vi "Measurement Logic.vi"() -> ()   [LabVIEW 2021, in "Waveform Mode_Channel Ganging.lvlib"]
uses:
  Waveform Mode_Channel Ganging.lvlib
  <vilib>/Plug-In SDKs/Measurements/Measure Call Context/Measure Call Context.lvclass
  Measurement Results.ctl
  Measurement Configuration.ctl
  shared/Ganging/controls/Power ON-Ganging.ctl
  shared/Single/controls/Power ON-Single.ctl
panel:
  in  "measurement configuration":T1={"Mode of operation"=enum."Power on the DUT", "Source voltage/current gain bandwidths"=[], "Source voltage/current compensation frequencies"=[], "Source voltage/current pole-zero ratios"=[], "Load voltage/current gain bandwidths"=[], "Load voltage/current compensation frequencies"=[], "Load voltage/current pole-zero ratios"=[], "Source enable/disable"=TRUE, "Load enable/disable"=FALSE, "Power ON/Source resource names"=[], "Load resource names"=[], "Power ON/Source voltage/current setpoints"=[], "Source source delays"=[], "Load voltage/current setpoints"=[], "Load source delays"=[], "Power ON/Source system configuration"=enum."Parallel", "Power ON/Source output function"=1006, "Source voltage/current level range"=20.0, "Power ON/Source sense"=1009, "Source limit symmetry"=enum."Asymmetric", "Power ON/Source current/voltage limit range"=25.0, "Source current/voltage limit low"=-0.6, "Source current/voltage limit high"=25.0, "Source aperture time"=0.01666, "Source transient response"=1038, "Load device voltage/current rating"=10.0, "Load system configuration"=enum."Parallel", "Load output function"=1007, "Load voltage/current level range"=80.0, "Load sense"=1009, "Load limit symmetry"=enum."Symmetric", "Load current/voltage limit range"=6.0, "Load current/voltage limit low"=0.0, "Load current/voltage limit high"=inf, "Load aperture time"=0.01666, "Load transient response"=1038, "Measurement timeout"=1.0} {"Measurement timeout" format="%.3p"; "Load device voltage/current rating" format="%#_6pA"; "Load voltage/current setpoints" format="%#_6p"; "Load output function" items=["DC Voltage"=1006, "DC Current"=1007, "Pulse Voltage"=1049, "Pulse Current"=1050]; "Load sense" items=["Local"=1008, "Remote"=1009]; "Load transient response" items=["Slow"=1041, "Normal"=1038, "Fast"=1039, "Custom"=1042]; "Load current/voltage limit high" format="%#_6p"; "Load current/voltage limit low" format="%#_6p"; "Load current/voltage limit range" format="%#_6p"; "Load voltage/current level range" format="%#_6p"; "Power ON/Source voltage/current setpoints" format="%#_6p"; "Power ON/Source output function" items=["DC Voltage"=1006, "DC Current"=1007, "Pulse Voltage"=1049, "Pulse Current"=1050]; "Power ON/Source sense" items=["Local"=1008, "Remote"=1009]; "Source transient response" items=["Slow"=1041, "Normal"=1038, "Fast"=1039, "Custom"=1042]; "Source current/voltage limit high" format="%#_6p"; "Source current/voltage limit low" format="%#_6p"; "Power ON/Source current/voltage limit range" format="%#_6p"; "Source voltage/current level range" format="%#_6p"}
  out "error out":errorcluster
  out "measurement results":T2
  out "measure call context out":refnum<class "Measure Call Context.lvclass">
  in  "measure call context in":refnum<class "Measure Call Context.lvclass">
  in  "error in":errorcluster
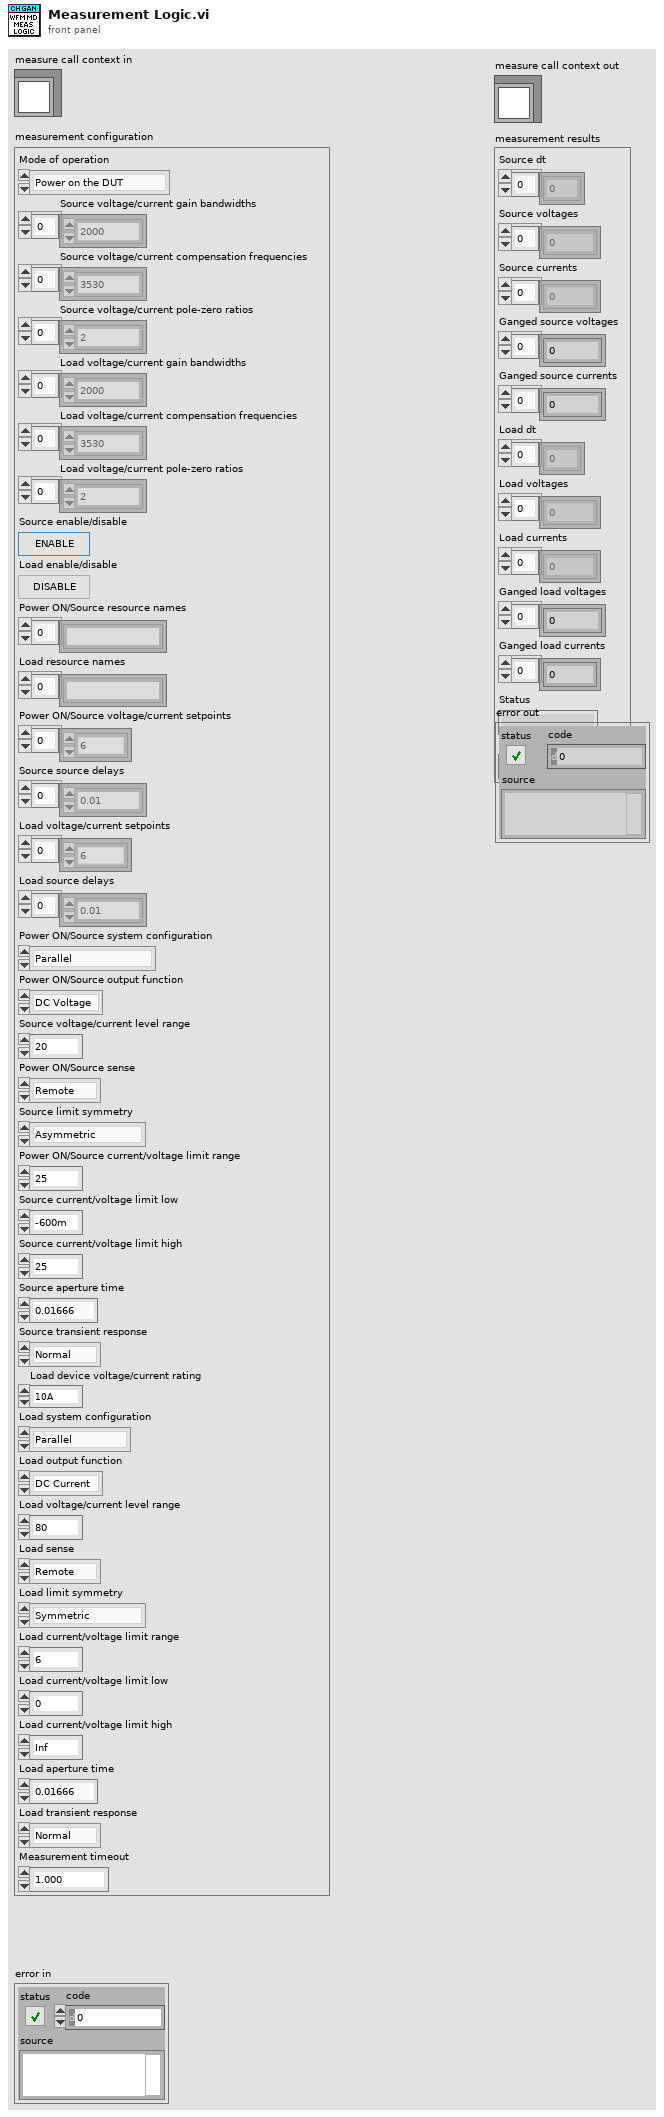
[diagram p1: front panel]
types:
  T1 = typedef "Waveform Mode_Channel Ganging.lvlib/Measurement Configuration.ctl" = cluster{"Mode of operation":enum32{"Power on the DUT", "Perform measurement", "Power off the DUT"}, "Source voltage/current gain bandwidths":dbl[], "Source voltage/current compensation frequencies":dbl[], "Source voltage/current pole-zero ratios":dbl[], "Load voltage/current gain bandwidths":dbl[], "Load voltage/current compensation frequencies":dbl[], "Load voltage/current pole-zero ratios":dbl[], "Source enable/disable":bool, "Load enable/disable":bool, "Power ON/Source resource names":string[], "Load resource names":string[], "Power ON/Source voltage/current setpoints":dbl[], "Source source delays":dbl[], "Load voltage/current setpoints":dbl[], "Load source delays":dbl[], "Power ON/Source system configuration":enum32{"Series", "Parallel", "Manual"}, "Power ON/Source output function":i32, "Source voltage/current level range":dbl, "Power ON/Source sense":i32, "Source limit symmetry":enum32{"Symmetric", "Asymmetric"}, "Power ON/Source current/voltage limit range":dbl, "Source current/voltage limit low":dbl, "Source current/voltage limit high":dbl, "Source aperture time":dbl, "Source transient response":i32, "Load device voltage/current rating":dbl, "Load system configuration":enum32{"Series", "Parallel", "Manual"}, "Load output function":i32, "Load voltage/current level range":dbl, "Load sense":i32, "Load limit symmetry":enum32{"Symmetric", "Asymmetric"}, "Load current/voltage limit range":dbl, "Load current/voltage limit low":dbl, "Load current/voltage limit high":dbl, "Load aperture time":dbl, "Load transient response":i32, "Measurement timeout":dbl}
  T2 = typedef "Waveform Mode_Channel Ganging.lvlib/Measurement Results.ctl" = cluster{"Source dt":dbl[], "Source voltages":dbl[], "Source currents":dbl[], "Ganged source voltages":dbl[], "Ganged source currents":dbl[], "Load dt":dbl[], "Load voltages":dbl[], "Load currents":dbl[], "Ganged load voltages":dbl[], "Ganged load currents":dbl[], "Status":string, "Eload status":string}
  T3 = enum32{"Power on the DUT", "Perform measurement", "Power off the DUT"}
  T4 = typedef "Power ON-Ganging.ctl" = cluster{"Master/single Resource name":string, "Slave resource name":string[], "System configuration":enum32{"Series", "Parallel", "Manual"}, "Output function":i32, "Voltage/current level":dbl, "Voltage/current limit":dbl, "Sense":i32}
  T5 = typedef "Power ON-Single.ctl" = cluster{"Voltage/current level":dbl, "Voltage/current limit":dbl, "Sense":i32, "Resource name":string, "Output function":i32}
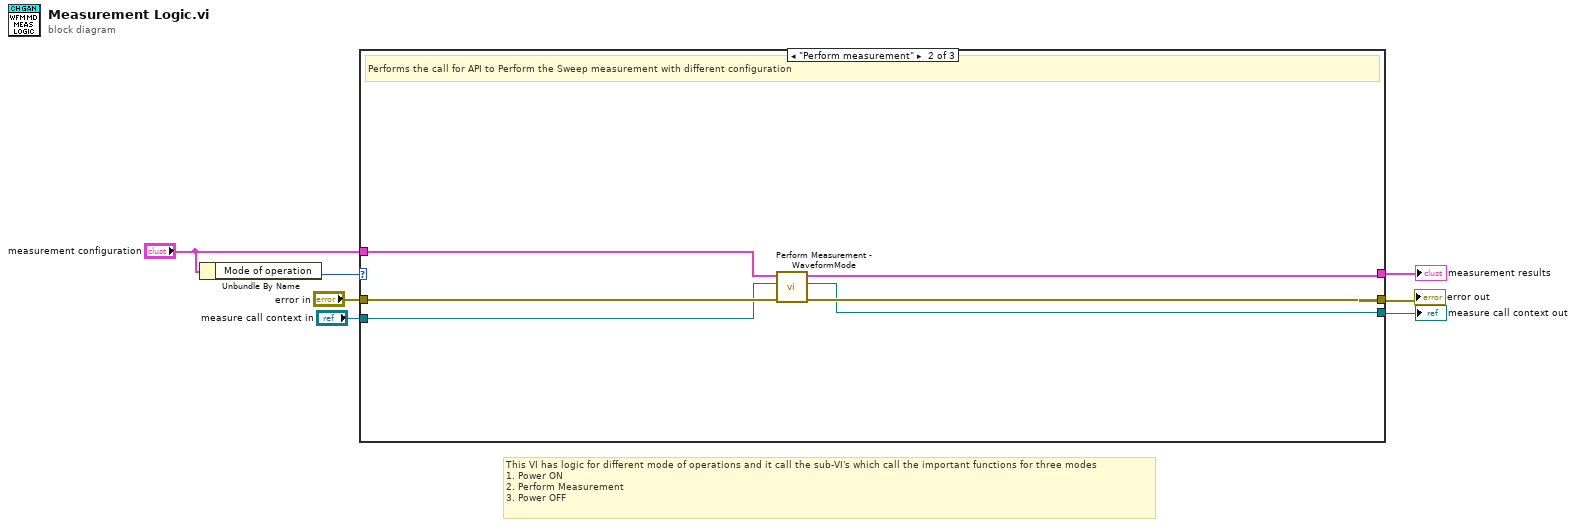
[diagram p0: block diagram]
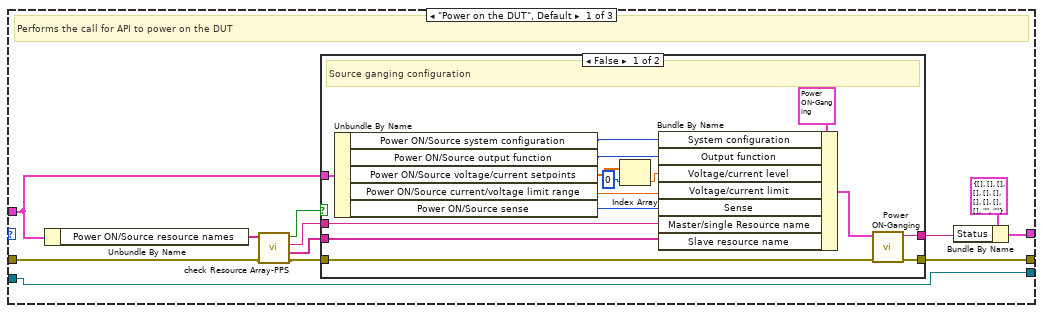
[diagram p2: hidden frame]
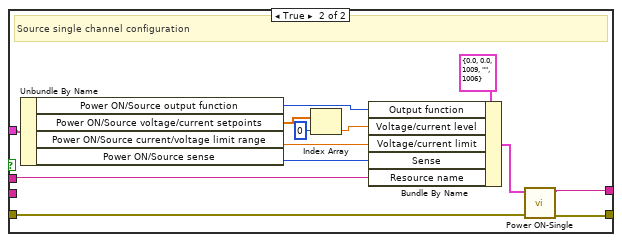
[diagram p3: hidden frame]
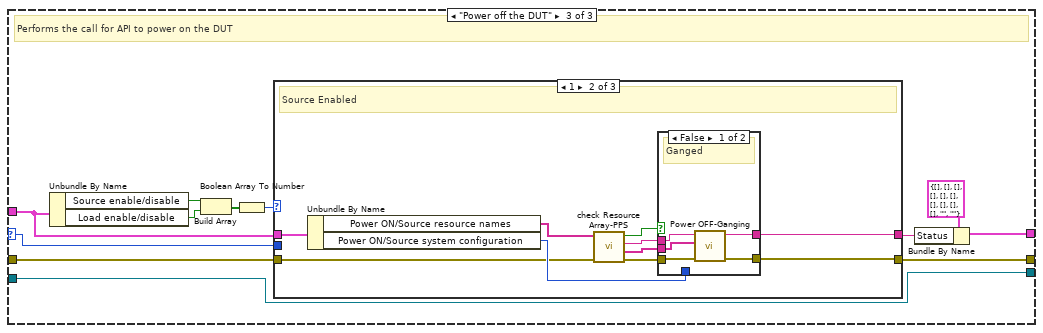
[diagram p4: hidden frame]
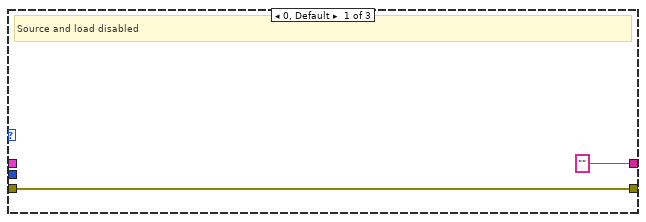
[diagram p5: hidden frame]
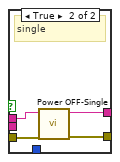
[diagram p6: hidden frame]
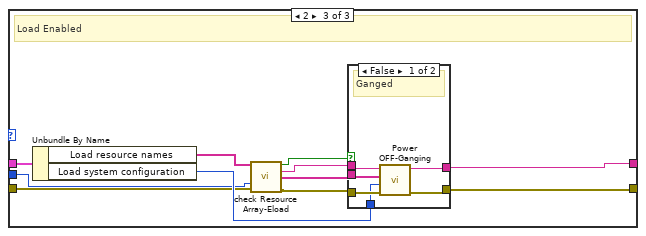
[diagram p7: hidden frame]
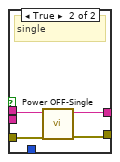
[diagram p8: hidden frame]
diagram:
  # "This VI has logic for different mode of operations and it call the sub-VI's which call the important functions for three modes\n1. Power ON\n2. Perform Measurement\n3. Power OFF"
  n1 = Unbundle By Name("measurement configuration") -> ("Mode of operation"=w2:T3)
  n2 = case shown="\"Perform measurement\"" w2 {
    selector: w2 -> [_ _ w54]
    tunnel: "error in" -> [w13 w53 w60]
    tunnel: "measure call context in" -> [w11 w50 w55]
    tunnel: [w11 w48 w55] -> w5
    tunnel: [w10 w49 w56] -> w4
    tunnel: "measurement configuration" -> [w12 w51 w59]
    tunnel: [w9 w52 w58] -> w3
    frame "Power on the DUT", Default {
      # "Performs the call for API to power on the DUT"
      n3 = Unbundle By Name(w12) -> ("Power ON/Source resource names"=w16:string[])
      n4 = call "check Resource Array-PPS.vi"("error in"=w13, "Resource names"=w16) -> ("error out"=w19:errorcluster, "Slave resource names"=w17:string[], "Single/Master resouce names"=w18:string, "Single or ganged configuration"=w15:bool)  [unwired: 6 in]
      n5 = case shown="False" w15 {
        tunnel: w19 -> [w27 w46]
        tunnel: [w28 w45] -> w9
        tunnel: w17 -> [w32 _]
        tunnel: w12 -> [w34 w47]
        tunnel: w18 -> [w33 w42]
        tunnel: [w29 w44] -> w14
        frame False {
          # "Source ganging configuration"
          n6 = Unbundle By Name(w34) -> ("Power ON/Source system configuration"=w26:enum32{"Series", "Parallel", "Manual"}, "Power ON/Source output function"=w25:i32, "Power ON/Source voltage/current setpoints"=w21:dbl[], "Power ON/Source current/voltage limit range"=w31:dbl, "Power ON/Source sense"=w30:i32)
          n7 = Index Array(array=w21, index=0) -> (element=w22:dbl)
          n8 = Bundle By Name(cluster=T4 {"Master/single Resource name"="", "Slave resource name"=[], "System configuration"=enum."Parallel", "Output function"=1006, "Voltage/current level"=0.0, "Voltage/current limit"=0.0, "Sense"=1009} ("Power ON"), "System configuration"=w26, "Output function"=w25, "Voltage/current level"=w22, "Voltage/current limit"=w31, "Sense"=w30, "Master/single Resource name"=w33, "Slave resource name"=w32) -> (w23:T4)
          n9 = call "Power ON-Ganging.vi"("error in"=w27, "Power ON"=w23) -> ("error out"=w28:errorcluster, "Status"=w29:string)  [unwired: 8 in]
        }
        frame True {
          # "Source single channel configuration"
          n10 = Unbundle By Name(w47) -> ("Power ON/Source output function"=w36:i32, "Power ON/Source voltage/current setpoints"=w40:dbl[], "Power ON/Source current/voltage limit range"=w38:dbl, "Power ON/Source sense"=w37:i32)
          n11 = Index Array(array=w40, index=0) -> (element=w39:dbl)
          n12 = Bundle By Name(cluster=T5 {"Voltage/current level"=0.0, "Voltage/current limit"=0.0, "Sense"=1009, "Resource name"="", "Output function"=1006} ("Power ON single"), "Output function"=w36, "Voltage/current level"=w39, "Voltage/current limit"=w38, "Sense"=w37, "Resource name"=w42) -> (w43:T5)
          n13 = call "Power ON-Single.vi"("error in"=w46, "Power ON single"=w43) -> ("error out"=w45:errorcluster, "Status"=w44:string)  [unwired: 8 in]
        }
      }
      n14 = Bundle By Name(cluster=T2 {"Source dt"=[], "Source voltages"=[], "Source currents"=[], "Ganged source voltages"=[], "Ganged source currents"=[], "Load dt"=[], "Load voltages"=[], "Load currents"=[], "Ganged load voltages"=[], "Ganged load currents"=[], "Status"="", "Eload status"=""} ("measurement results"), "Status"=w14) -> (w10:T2)
    }
    frame "Perform measurement" {
      # "Performs the call for API to Perform the Sweep measurement with different configuration"
      n15 = call "Perform Measurement - WaveformMode.vi"("error in"=w53, "Measure Call Context in"=w50, "measurement configuration"=w51) -> ("error out"=w52:errorcluster, "Measure Call Context out"=w48:refnum<class "Measure Call Context.lvclass">, "Measurement Results"=w49:T2)  [unwired: 6 in]
    }
    frame "Power off the DUT" {
      # "Performs the call for API to power on the DUT"
      n16 = Unbundle By Name(w59) -> ("Source enable/disable"=w65:bool, "Load enable/disable"=w64:bool)
      n17 = Build Array(w65, w64) -> (w63:bool[])
      n18 = Boolean Array To Number(Boolean array=w63) -> (number=w62:u32)
      n19 = case shown="1" w62 {
        tunnel: w59 -> [_ w77 w97]
        tunnel: w60 -> [w67 w72 w93]
        tunnel: [w67 w76 w96] -> w58
        tunnel: ["" ("Status") w74 w95] -> w61
        tunnel: w54 -> [_ _ w87]
        frame 0, Default {
          # "Source and load disabled"
        }
        frame 1 {
          # "Source Enabled"
          n20 = Unbundle By Name(w77) -> ("Power ON/Source resource names"=w73:string[], "Power ON/Source system configuration"=w75:enum32{"Series", "Parallel", "Manual"})
          n21 = call "check Resource Array-PPS.vi"("error in"=w72, "Resource names"=w73) -> ("error out"=w71:errorcluster, "Slave resource names"=w68:string[], "Single/Master resouce names"=w69:string, "Single or ganged configuration"=w70:bool)  [unwired: 6 in]
          n22 = case shown="False" w70 {
            tunnel: w71 -> [w82 w84]
            tunnel: [w78 w85] -> w76
            tunnel: [w81 w86] -> w74
            tunnel: w75 -> [_ _]
            tunnel: w69 -> [w80 w83]
            tunnel: w68 -> [w79 _]
            frame False {
              # "Ganged"
              n23 = call "Power OFF-Ganging.vi"("error in"=w82, "Slave resource names"=w79, "Master resouce name"=w80) -> ("error out"=w78:errorcluster, "Status"=w81:string)  [unwired: 7 in]
            }
            frame True {
              # "single"
              n24 = call "Power OFF-Single.vi"("error in (no error)"=w84, "Resource name"=w83) -> ("error out"=w85:errorcluster, "Status"=w86:string)  [unwired: 8 in]
            }
          }
        }
        frame 2 {
          # "Load Enabled"
          n25 = Unbundle By Name(w97) -> ("Load resource names"=w89:string[], "Load system configuration"=w94:enum32{"Series", "Parallel", "Manual"})
          n26 = call "check Resource Array-Eload.vi"("Resource names"=w89, "Mode of operation"=w87, "error in"=w93) -> ("Single or ganged configuration"=w92:bool, "Single/Master resouce name"=w91:string, "Slave resource names"=w90:string[], "error out"=w88:errorcluster)  [unwired: 8 in, 1 out]
          n27 = case shown="False" w92 {
            tunnel: w88 -> [w103 w106]
            tunnel: [w98 w104] -> w96
            tunnel: [w102 w105] -> w95
            tunnel: w91 -> [w101 w107]
            tunnel: w90 -> [w100 _]
            tunnel: w94 -> [w99 _]
            frame False {
              # "Ganged"
              n28 = call "Power OFF-Ganging.vi"("error in"=w103, "Ganged Config"=w99, "Slave resource names"=w100, "Master resouce name"=w101) -> ("error out"=w98:errorcluster, "Status"=w102:string)  [unwired: 6 in]
            }
            frame True {
              # "single"
              n29 = call "Power OFF-Single.vi"("error in (no error)"=w106, "Resource name"=w107) -> ("error out"=w104:errorcluster, "Status"=w105:string)  [unwired: 8 in]
            }
          }
        }
      }
      n30 = Bundle By Name(cluster=T2 {"Source dt"=[], "Source voltages"=[], "Source currents"=[], "Ganged source voltages"=[], "Ganged source currents"=[], "Load dt"=[], "Load voltages"=[], "Load currents"=[], "Ganged load voltages"=[], "Ganged load currents"=[], "Status"="", "Eload status"=""} ("measurement results"), "Status"=w61) -> (w56:T2)
    }
  }
  "measure call context out" <- w5
  "measurement results" <- w4
  "error out" <- w3
